vi "Finish.vi"   [LabVIEW 2018]
doc: "This VI is called just before exiting. It is expected to close I/O refnum, save collected data, etc."
uses:
  <vilib>/Rock Robotics/WPI/Utilities/WPI_GetSetVariantRefNum.vi
types:
  T1 = typedef "WPI_JoystickDevRef.ctl" = cluster{"Device":T2}
  T2 = typedef "WPI_JoystickDeviceEnum.ctl" = enum16{"USB 0", "USB 1", "USB 2", "USB 3", "USB 4", "USB 5"}
  T3 = typedef "WPI_SolenoidDevRef.ctl" = cluster{"DevStatus":errorcluster, "Pneumatics Control Module":u8, "Forward Solenoid Channel":T4, "Reverse Solenoid Channel":T4}
  T4 = typedef "WPI_SolenoidChannel.ctl" = enum8{"Solenoid 0", "Solenoid 1", "Solenoid 2", "Solenoid 3", "Solenoid 4", "Solenoid 5", "Solenoid 6", "Solenoid 7", "Invalid"}
  T5 = typedef "WPI_CompressorDevRef.ctl" = cluster{"DevStatus":errorcluster, "Pneumatics Control Module":u8}
  T6 = typedef "WPI_SwitchDevRef.ctl" = cluster{"DevStatus":errorcluster, "DIO Channel":T7, "CntIndex":T8, "Normally Closed":bool}
  T7 = typedef "FPGA_DIOChannel.ctl" = enum8{"DIO 0", "DIO 1", "DIO 2", "DIO 3", "DIO 4", "DIO 5", "DIO 6", "DIO 7", "DIO 8", "DIO 9", "DIO MXP 0", "DIO MXP 1", "DIO MXP 2", "DIO MXP 3", "DIO MXP 4", "DIO MXP 5", "DIO MXP 6", "DIO MXP 7", "DIO MXP 8", "DIO MXP 9", "DIO MXP 10", "DIO MXP 11", "DIO MXP 12", "DIO MXP 13", "DIO MXP 14", "DIO MXP 15", "SPI Port CS1", "SPI Port CS2", "SPI Port CS3", "SPI Port MISO", "SPI Port MOSI", "Invalid"}
  T8 = typedef "FPGA_CounterCtrSystemIndex.ctl" = enum8{"Ctr 0", "Ctr 1", "Ctr 2", "Ctr 3", "Ctr 4", "Ctr 5", "Ctr 6", "Ctr 7", "Invalid"}
  T9 = typedef "WPI_MotorControlDeviceRef.ctl" = cluster{"DeviceStatus":errorcluster, "Type":T10, "PWM":cluster{"PWM Channel":T11, "DeadBand":T12}, "CAN":cluster{"Device Number":u8, "SetOutput VI Ref":variant, "GetOutput VI Ref":variant, "Enable VI Ref":variant, "Disable VI Ref":variant, "Data":variant}, "Invert":bool, "DIO PWM":cluster{"PWM \"Enable\" Channel":T11, "DIOChannel":T7, "PWM Rate":dbl}}
  T10 = typedef "WPI_MotorControlType.ctl" = enum16{"PWM", "CAN", "DIO PWM"}
  T11 = typedef "FPGA_DIOPWMChannel.ctl" = enum8{"PWM 0", "PWM 1", "PWM 2", "PWM 3", "PWM 4", "PWM 5", "PWM 6", "PWM 7", "PWM 8", "PWM 9", "PWM MXP 0", "PWM MXP 1", "PWM MXP 2", "PWM MXP 3", "PWM MXP 4", "PWM MXP 5", "PWM MXP 6", "PWM MXP 7", "PWM MXP 8", "PWM MXP 9", "Invalid"}
  T12 = typedef "WPI_PWMDeadband.ctl" = cluster{"Name":string, "maxPositivePwm":i32, "minPositivePwm":i32, "centerPwm":i32, "maxNegativePwm":i32, "minNegativePwm":i32, "angularRange":u16}
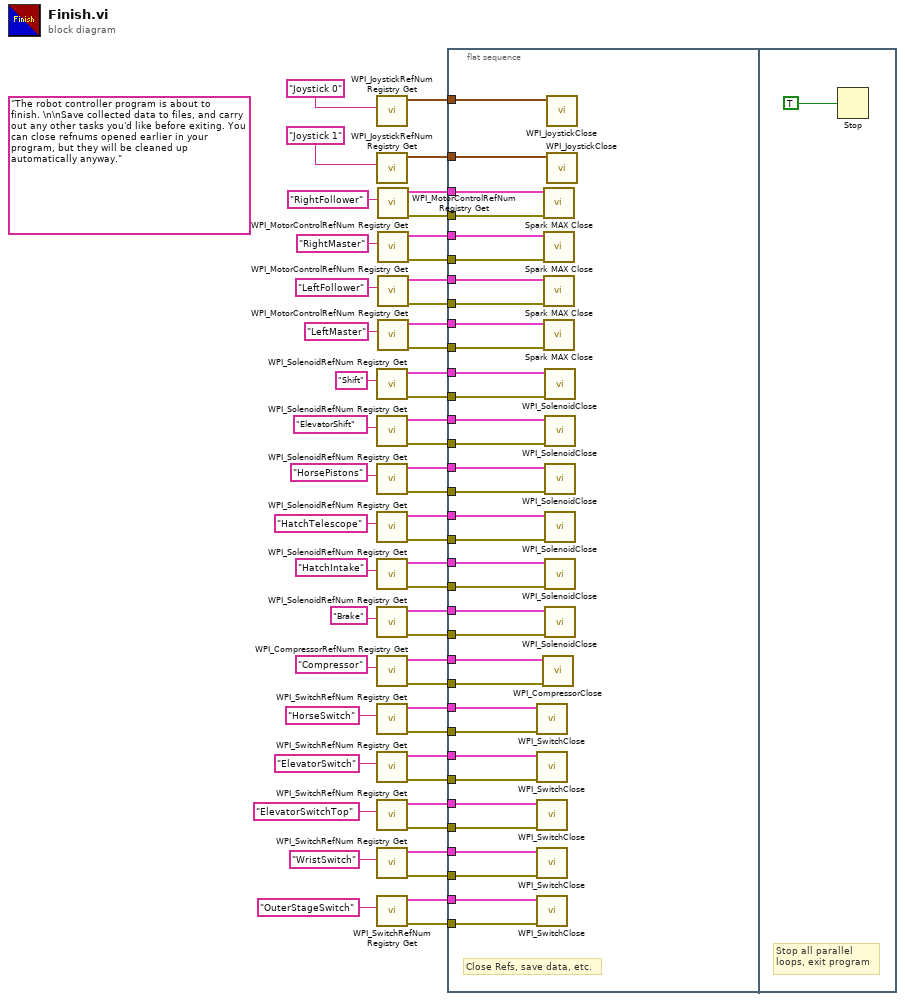
[diagram p0: block diagram]
diagram:
  (unwired) "The robot controller program is about to finish. \n\nSave collected data to files, and carry out any other tasks you'd like before exiting. You can close refnums opened earlier in your program, but they will be cleaned up automatically anyway."
  n1 = call <vilib>:"WPI_JoystickRefNum Registry Get.vi"("refnum name"="Joystick 0") -> ("JoystickDevRef"=w51:T1)  [unwired: 1 in, 9 out]
  n2 = call <vilib>:"WPI_JoystickRefNum Registry Get.vi"("refnum name"="Joystick 1") -> ("JoystickDevRef"=w26:T1)  [unwired: 1 in, 9 out]
  n3 = call <vilib>:"WPI_SolenoidRefNum Registry Get.vi"("refnum name"="Shift") -> ("error out"=w37:errorcluster, "SolenoidDevRef"=w38:T3)  [unwired: 9 in]
  n4 = call <vilib>:"WPI_SolenoidRefNum Registry Get.vi"("refnum name"="ElevatorShift") -> ("error out"=w31:errorcluster, "SolenoidDevRef"=w30:T3)  [unwired: 9 in]
  n5 = call <vilib>:"WPI_SolenoidRefNum Registry Get.vi"("refnum name"="HorsePistons") -> ("error out"=w34:errorcluster, "SolenoidDevRef"=w35:T3)  [unwired: 9 in]
  n6 = call <vilib>:"WPI_SolenoidRefNum Registry Get.vi"("refnum name"="HatchTelescope") -> ("error out"=w2:errorcluster, "SolenoidDevRef"=w1:T3)  [unwired: 9 in]
  n7 = call <vilib>:"WPI_SolenoidRefNum Registry Get.vi"("refnum name"="HatchIntake") -> ("error out"=w8:errorcluster, "SolenoidDevRef"=w9:T3)  [unwired: 9 in]
  n8 = call <vilib>:"WPI_SolenoidRefNum Registry Get.vi"("refnum name"="Brake") -> ("error out"=w5:errorcluster, "SolenoidDevRef"=w4:T3)  [unwired: 9 in]
  n9 = call <vilib>:"WPI_CompressorRefNum Registry Get.vi"("refnum name"="Compressor") -> ("error out"=w28:errorcluster, "CompressorDevRef"=w29:T5)  [unwired: 9 in]
  n10 = call <vilib>:"WPI_SwitchRefNum Registry Get.vi"("refnum name"="HorseSwitch") -> ("error out"=w22:errorcluster, "SwitchDevRef"=w23:T6)  [unwired: 9 in]
  n11 = call <vilib>:"WPI_SwitchRefNum Registry Get.vi"("refnum name"="ElevatorSwitch") -> ("error out"=w21:errorcluster, "SwitchDevRef"=w20:T6)  [unwired: 9 in]
  n12 = call <vilib>:"WPI_SwitchRefNum Registry Get.vi"("refnum name"="ElevatorSwitchTop") -> ("error out"=w16:errorcluster, "SwitchDevRef"=w17:T6)  [unwired: 9 in]
  n13 = call <vilib>:"WPI_SwitchRefNum Registry Get.vi"("refnum name"="WristSwitch") -> ("error out"=w15:errorcluster, "SwitchDevRef"=w14:T6)  [unwired: 9 in]
  n14 = call <vilib>:"WPI_SwitchRefNum Registry Get.vi"("refnum name"="OuterStageSwitch") -> ("error out"=w10:errorcluster, "SwitchDevRef"=w11:T6)  [unwired: 9 in]
  n15 = call <vilib>:"WPI_MotorControlRefNum Registry Get.vi"("refnum name"="RightFollower") -> ("error out"=w49:errorcluster, "MotorControlDevRef"=w50:T9)  [unwired: 9 in]
  n16 = call <vilib>:"WPI_MotorControlRefNum Registry Get.vi"("refnum name"="RightMaster") -> ("error out"=w46:errorcluster, "MotorControlDevRef"=w45:T9)  [unwired: 9 in]
  n17 = call <vilib>:"WPI_MotorControlRefNum Registry Get.vi"("refnum name"="LeftFollower") -> ("error out"=w40:errorcluster, "MotorControlDevRef"=w39:T9)  [unwired: 9 in]
  n18 = call <vilib>:"WPI_MotorControlRefNum Registry Get.vi"("refnum name"="LeftMaster") -> ("error out"=w43:errorcluster, "MotorControlDevRef"=w44:T9)  [unwired: 9 in]
  n19 = flat-sequence {
    tunnel: w51 -> [w86]
    tunnel: w50 -> [w85]
    tunnel: w49 -> [w84]
    tunnel: w45 -> [w82]
    tunnel: w46 -> [w83]
    tunnel: w39 -> [w78]
    tunnel: w40 -> [w79]
    tunnel: w44 -> [w81]
    tunnel: w43 -> [w80]
    tunnel: w38 -> [w77]
    tunnel: w37 -> [w76]
    tunnel: w30 -> [w72]
    tunnel: w31 -> [w73]
    tunnel: w35 -> [w75]
    tunnel: w34 -> [w74]
    tunnel: w29 -> [w71]
    tunnel: w28 -> [w70]
    tunnel: w26 -> [w69]
    tunnel: w23 -> [w68]
    tunnel: w22 -> [w67]
    tunnel: w20 -> [w65]
    tunnel: w21 -> [w66]
    tunnel: w17 -> [w64]
    tunnel: w16 -> [w63]
    tunnel: w14 -> [w61]
    tunnel: w15 -> [w62]
    tunnel: w11 -> [w60]
    tunnel: w10 -> [w59]
    tunnel: w1 -> [w53]
    tunnel: w2 -> [w54]
    tunnel: w9 -> [w58]
    tunnel: w8 -> [w57]
    tunnel: w4 -> [w55]
    tunnel: w5 -> [w56]
    frame #0 {
      # "Close Refs, save data, etc."
      n20 = call <vilib>:"WPI_SwitchClose.vi"("error in (no error)"=w67, "SwitchDevRef"=w68) -> ()  [unwired: 9 in, 1 out]
      n21 = call <vilib>:"WPI_SwitchClose.vi"("error in (no error)"=w66, "SwitchDevRef"=w65) -> ()  [unwired: 9 in, 1 out]
      n22 = call <vilib>:"WPI_SwitchClose.vi"("error in (no error)"=w63, "SwitchDevRef"=w64) -> ()  [unwired: 9 in, 1 out]
      n23 = call <vilib>:"WPI_SwitchClose.vi"("error in (no error)"=w62, "SwitchDevRef"=w61) -> ()  [unwired: 9 in, 1 out]
      n24 = call <vilib>:"WPI_SwitchClose.vi"("error in (no error)"=w59, "SwitchDevRef"=w60) -> ()  [unwired: 9 in, 1 out]
      n25 = call <vilib>:"WPI_CompressorClose.vi"("error in (no error)"=w70, "CompressorDevRef"=w71) -> ()  [unwired: 9 in, 1 out]
      n26 = call <vilib>:"Spark MAX Close.vi"("error in"=w84, "MotorControlDeviceRef"=w85) -> ()  [unwired: 9 in, 1 out]
      n27 = call <vilib>:"Spark MAX Close.vi"("error in"=w83, "MotorControlDeviceRef"=w82) -> ()  [unwired: 9 in, 1 out]
      n28 = call <vilib>:"Spark MAX Close.vi"("error in"=w79, "MotorControlDeviceRef"=w78) -> ()  [unwired: 9 in, 1 out]
      n29 = call <vilib>:"Spark MAX Close.vi"("error in"=w80, "MotorControlDeviceRef"=w81) -> ()  [unwired: 9 in, 1 out]
      n30 = call <vilib>:"WPI_SolenoidClose.vi"("error in (no error)"=w76, "SolenoidDevRef"=w77) -> ()  [unwired: 9 in, 1 out]
      n31 = call <vilib>:"WPI_SolenoidClose.vi"("error in (no error)"=w73, "SolenoidDevRef"=w72) -> ()  [unwired: 9 in, 1 out]
      n32 = call <vilib>:"WPI_SolenoidClose.vi"("error in (no error)"=w74, "SolenoidDevRef"=w75) -> ()  [unwired: 9 in, 1 out]
      n33 = call <vilib>:"WPI_SolenoidClose.vi"("error in (no error)"=w54, "SolenoidDevRef"=w53) -> ()  [unwired: 9 in, 1 out]
      n34 = call <vilib>:"WPI_SolenoidClose.vi"("error in (no error)"=w57, "SolenoidDevRef"=w58) -> ()  [unwired: 9 in, 1 out]
      n35 = call <vilib>:"WPI_SolenoidClose.vi"("error in (no error)"=w56, "SolenoidDevRef"=w55) -> ()  [unwired: 9 in, 1 out]
      n36 = call <vilib>:"WPI_JoystickClose.vi"("JoystickDevRef"=w86) -> ()  [unwired: 11 out]
      n37 = call <vilib>:"WPI_JoystickClose.vi"("JoystickDevRef"=w69) -> ()  [unwired: 11 out]
    }
    frame #1 {
      # "Stop all parallel\nloops, exit program"
      n38 = Stop(stop? (T)=TRUE ("Quit")) -> ()
    }
  }
